vi "Add Activity to File (No DIT).vi"(8 "error out":errorcluster, 9 "Sample ID":string, 10 "date/time string":string, 11 "Activity Log filepath":path) -> (0 "error in (no error)":errorcluster)   [LabVIEW 2013]
doc: "Appends an activity string to the Activity Log file."
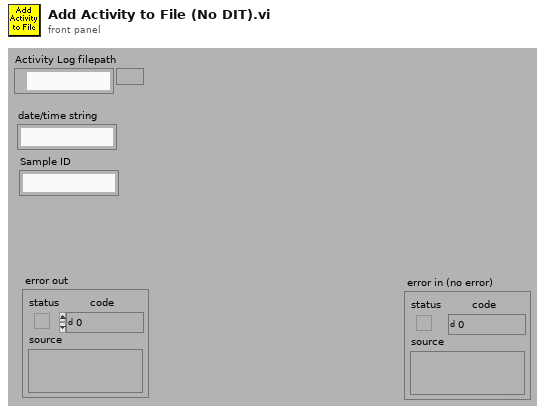
[diagram p1: front panel]
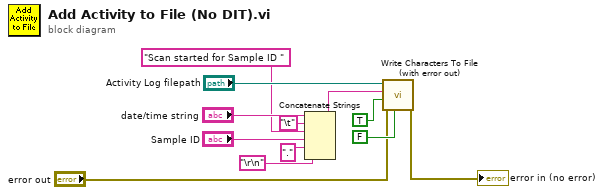
[diagram p0: block diagram]
diagram:
  n1 = Concatenate Strings("date/time string", "\t", "Scan started for Sample ID " ("string"), "Sample ID", "." ("string"), "\r\n") -> (w12:string)
  n2 = call "Write Characters To File (with error out).vi"("advisory dialog? (display:T)"=FALSE, "error in (no error)"="error out", "append to file? (new file:F)"=TRUE, "character string"=w12, "file path (dialog if empty)"="Activity Log filepath") -> ("error out"=→"error in (no error)":errorcluster)  [unwired: 5 in, 1 out]
